vi "thermistor_reduced_R.vi"() -> ()   [LabVIEW 2018]
uses:
  <vilib>/rvi/FXPMathLib/FxpMul/XNode/nifxpmath_Multiplier.xnode
  <vilib>/rvi/FXPMathLib/FxpDiv/XNode/nifxpmath_Div.xnode
  <vilib>/rvi/FXPMathLib/sim/FxpSim.dll
  <vilib>/rvi/FXPMathLib/FxpDiv/simVIs/DllFxpDivTemp_sub.vi
  <vilib>/rvi/FXPMathLib/FxpDiv/subVIs/nifxpmath_Div_SimConfig.ctl
  <vilib>/rvi/FXPMathLib/FxpSub/XNode/nifxpmath_Sub.xnode
panel:
  out "output valid":bool
  out "R^~":fxp<+/-,64,34>
  in  "ready for output (T)":bool=TRUE
  in  "input valid":bool=TRUE
  in  "1/R_inf":fxp<+/-,32,16>
  in  "V":fxp<+,20,4>
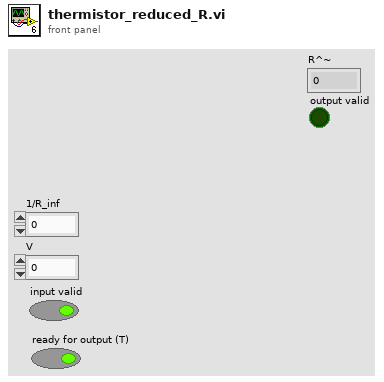
[diagram p1: front panel]
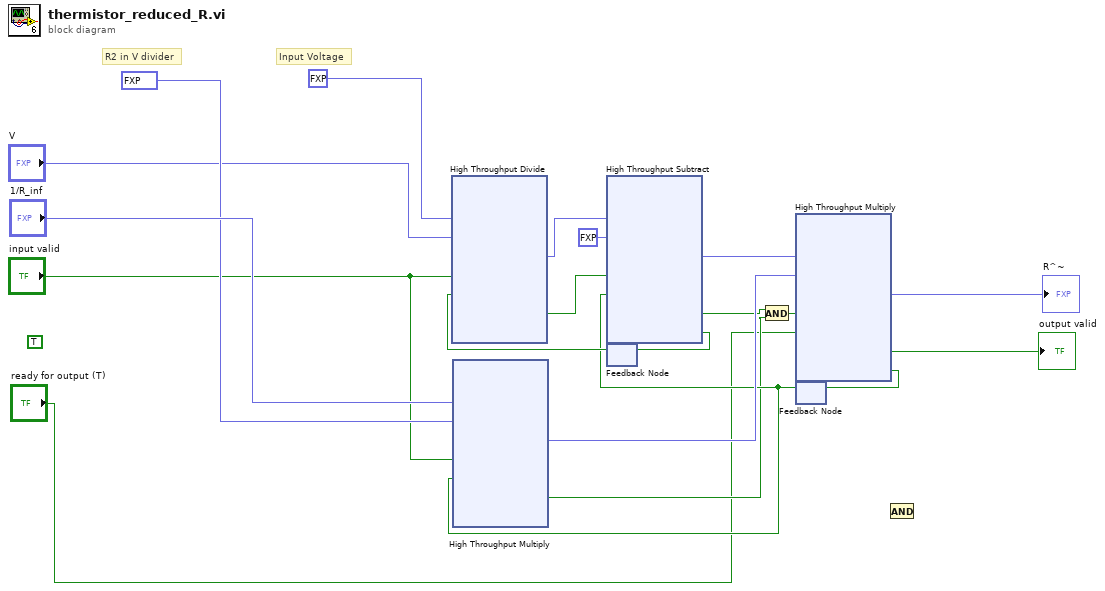
[diagram p0: block diagram]
diagram:
  (unwired) TRUE
  # "Input Voltage"
  # "R2 in V divider"
  n1 = feedback #1() -> (w12:bool)  [unwired: 1 in]
  n2 = xnode "High Throughput Divide"("x"=fxp<+,4,4> 12.0, "y"="V", "input valid"="input valid", "ready for output (T)"=w12) -> ("x/y"=w16:fxp<+,20,4>, "output valid"=w14:bool)  [unwired: 1 out]
  n3 = feedback #2() -> (w7:bool)  [unwired: 1 in]
  n4 = xnode "High Throughput Multiply"("x"="1/R_inf", "y"=fxp<+,14,14> 10000.0, "input valid"="input valid", "ready for output (T)"=w7) -> ("x*y"=w10:fxp<+/-,46,30>, "output valid"=w4:bool)  [unwired: 1 out]
  n5 = xnode "High Throughput Subtract"("x"=w16, "y"=fxp<+,1,1> 1.0, "input valid"=w14, "ready for output (T)"=w7) -> ("x-y"=w9:fxp<+,20,4>, "output valid"=w5:bool, "ready for input"=w13:bool)
  n6 = feedback-in #1(w13) -> ()
  n7 = And(x=w5, y=w4) -> (x .and. y?=w6:bool)
  n8 = xnode "High Throughput Multiply"("x"=w9, "y"=w10, "input valid"=w6, "ready for output (T)"="ready for output (T)") -> ("x*y"=→"R^~":fxp<+/-,64,34>, "output valid"=→"output valid":bool, "ready for input"=w8:bool)
  n9 = feedback-in #2(w8) -> ()
  n10 = And() -> ()  [unwired: 2 in, 1 out]
